vi "Main.vi"(8 "error in":errorcluster, 11 "ooxxMeter in":refnum<class "ooxxMeter.lvclass">) -> (0 "error out":errorcluster, 3 "ooxxMeter out":refnum<class "ooxxMeter.lvclass">)   [LabVIEW 2024, in "ooxxMeter.lvclass"]
doc: "The <b>Queued Message Handler</b> of the Worker that owns this VI."
uses:
  ooxxMeter.lvclass
  Initialization Data.ctl
  Response Cases.ctl
  <vilib>/addons/_Workers/Library/Case Label.ctl
  ooxxMeter.lvclass/ooxxMeter.ctl
  rql_MeterReadLoop.ctl
  rql_UpdatePanelDisplay.ctl
  rwr_ReadMeterValueNow.ctl
  rwr_ReadMeterValueNow Reply.ctl
  rqp_ReadValueAvg.ctl
  rsp_ReturnValueAvg.ctl
  <vilib>/numeric/Random Number (Range) DBL.vi
  20c30a35-eba6-49d0-a73b-0a0021e1c17a.vi
  <vilib>/Analysis/baseanly.llb/Mean (DBL).vi
  <vilib>/addons/_Workers/Library/Workers.lvlib
  <vilib>/Analysis/NI_AALBase.lvlib
panel:
  out "Meter":dbl(knob) scale=0.0..100.0
  out "ProgressBar":u8(slide) scale=0.0..100.0
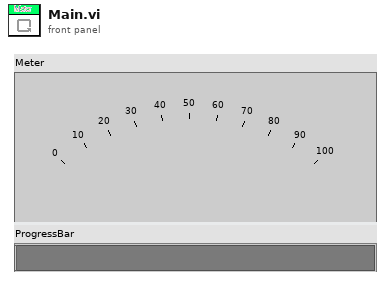
[diagram p1: front panel]
types:
  T1 = typedef "ooxxMeter.lvclass/Initialization Data.ctl" = cluster{"Response Cases":T2}
  T2 = typedef "ooxxMeter.lvclass/Response Cases.ctl" = cluster{"Placeholder - Can be deleted":string, "ReturnValueAvg":T3}
  T3 = typedef "Workers.lvlib/Case Label.ctl" = string
  T4 = typedef "ooxxMeter.lvclass/rql_MeterReadLoop.ctl" = cluster{"String":string}
  T5 = typedef "ooxxMeter.lvclass/rql_UpdatePanelDisplay.ctl" = cluster{"String":string}
  T6 = typedef "ooxxMeter.lvclass/rwr_ReadMeterValueNow Reply.ctl" = cluster{"String":string, "MeterValue":dbl}
  T7 = typedef "ooxxMeter.lvclass/rwr_ReadMeterValueNow.ctl" = cluster{"String":string}
  T8 = typedef "ooxxMeter.lvclass/rsp_ReturnValueAvg.ctl" = cluster{"String":string, "ValueAvg":dbl}
  T9 = typedef "ooxxMeter.lvclass/rqp_ReadValueAvg.ctl" = cluster{"String":string}
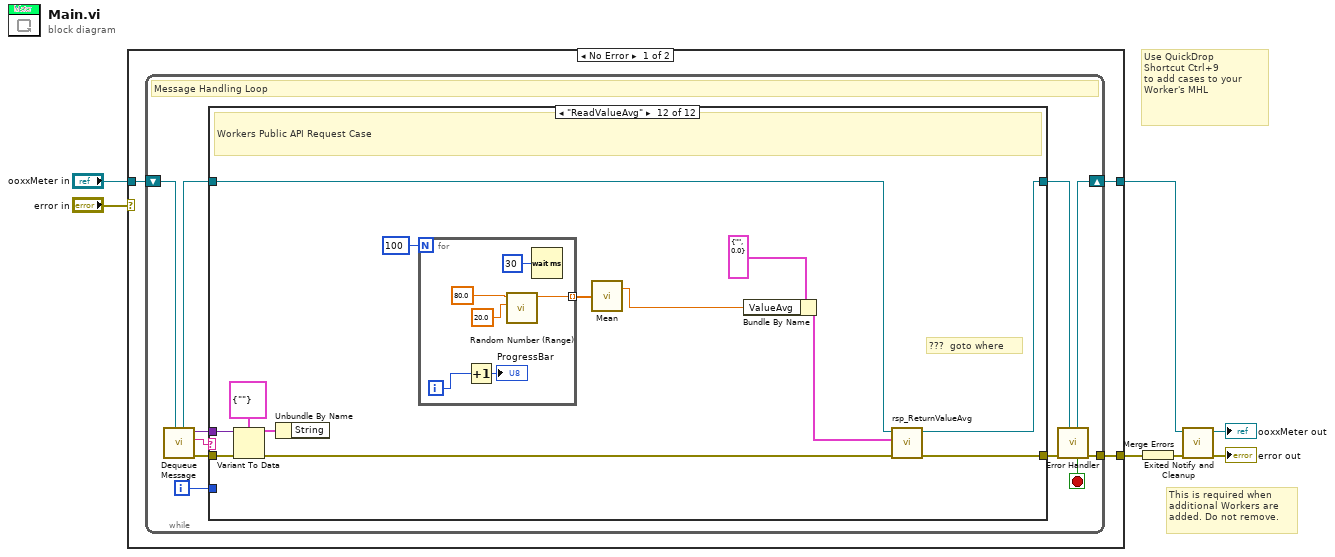
[diagram p0: block diagram]
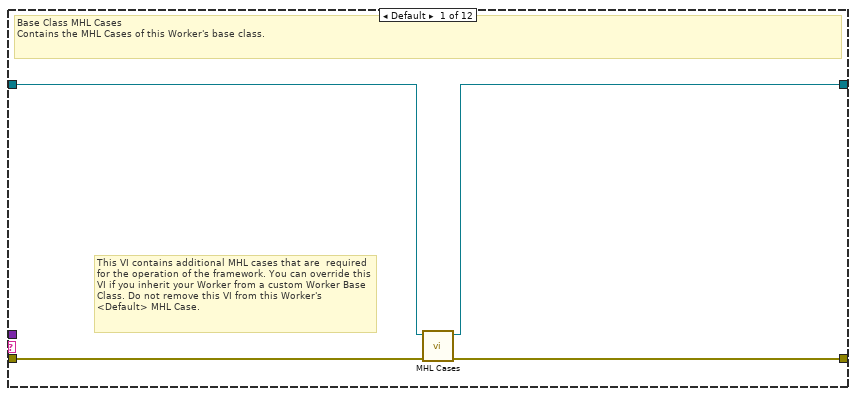
[diagram p2: hidden frame]
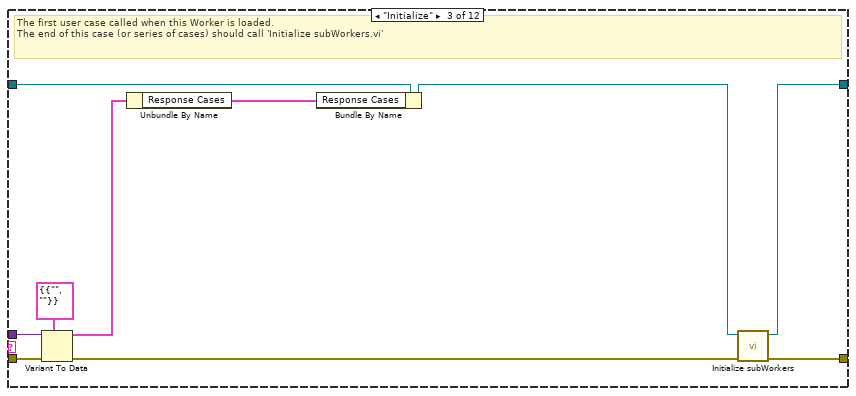
[diagram p4: hidden frame]
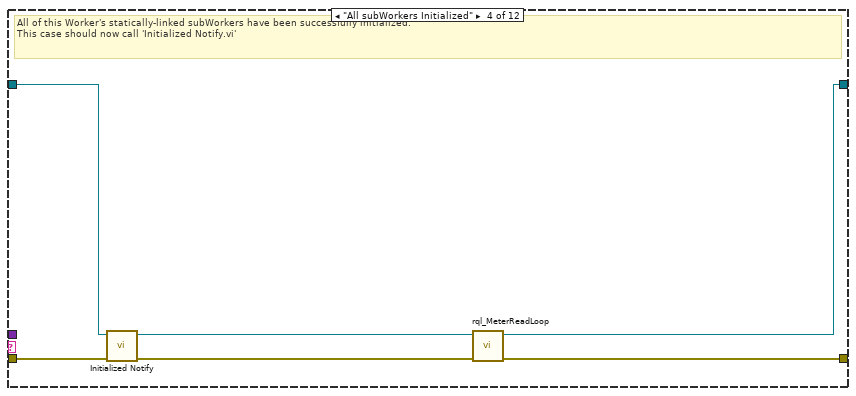
[diagram p5: hidden frame]
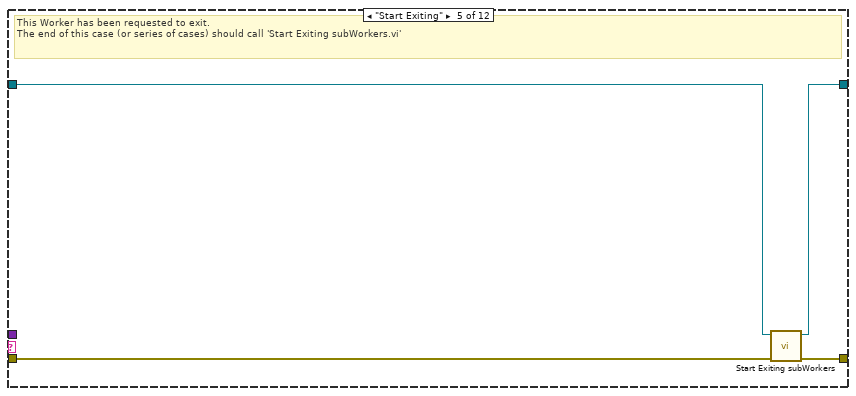
[diagram p6: hidden frame]
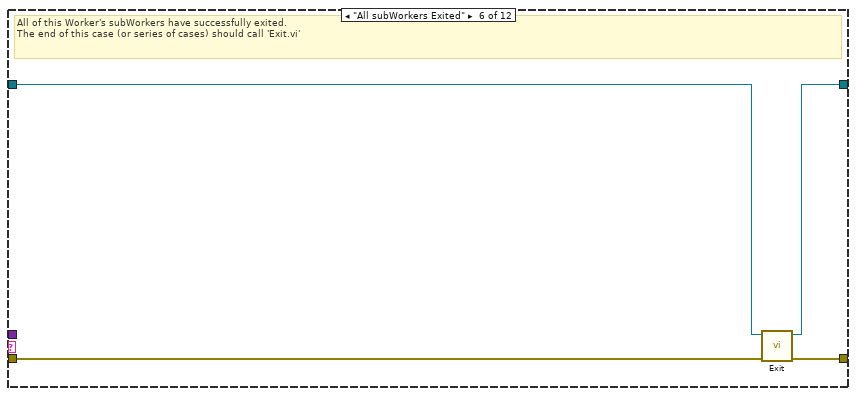
[diagram p7: hidden frame]
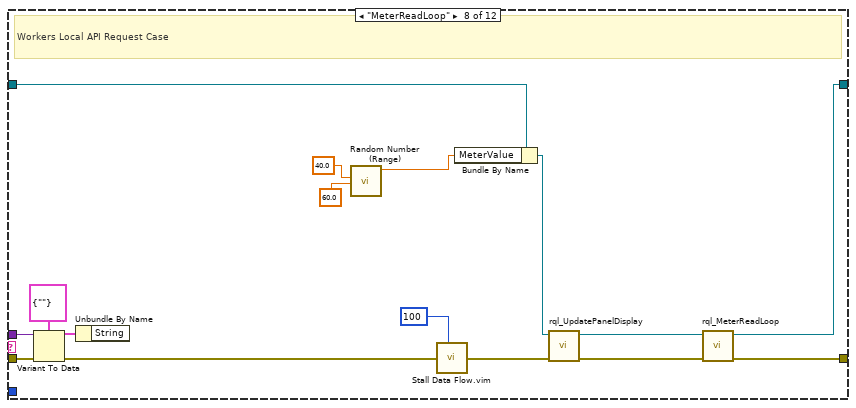
[diagram p9: hidden frame]
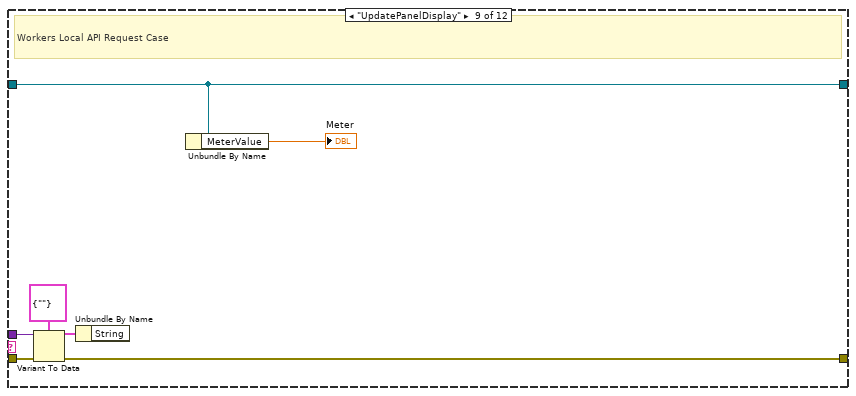
[diagram p10: hidden frame]
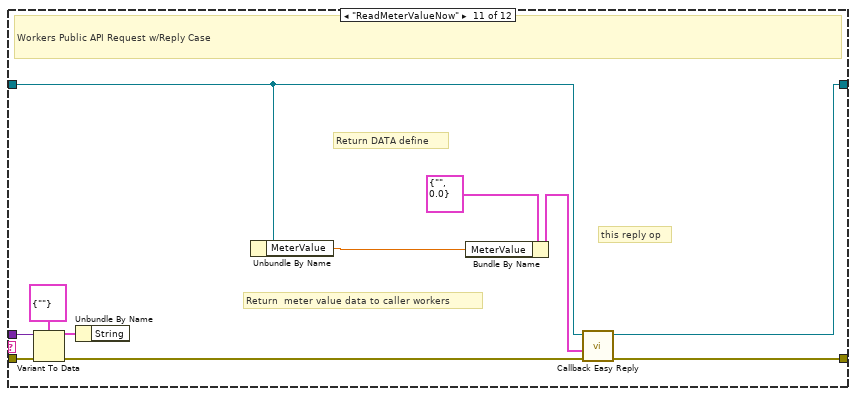
[diagram p12: hidden frame]
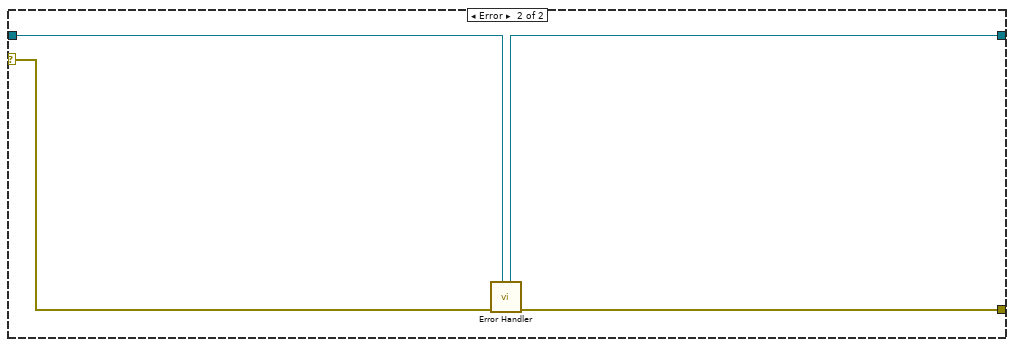
[diagram p13: hidden frame]
diagram:
  # "Use QuickDrop\nShortcut Ctrl+9\nto add cases to your\nWorker's MHL"
  # "This is required when additional Workers are added. Do not remove."
  n1 = case shown="No Error" "error in" {
    tunnel: "ooxxMeter in" -> [w8 w110]
    tunnel: [w10 w111] -> w6
    tunnel: [w9 w109] -> w7
    selector: "error in" -> [_ w112]
    frame No Error {
      n2 = while {
        shift-right: [w19] -> w9
        shift-left: w8 -> [w21]
        tunnel: [w20] -> w10
        i -> [w12]
        stop <- w13 stop-if-true
        # "Message Handling Loop"
        n3 = call-dynamic "Dequeue Message.vi"("Worker"=w21) -> ("error out"=w18:errorcluster, "Case out"=w14:string, "Data out"=w11:variant, "Worker out"=w16:refnum<class "ooxxMeter.lvclass">)  [unwired: 6 in, 1 out]
        n4 = case "Worker MHL Case Structure (DO NOT CHANGE LABEL NAME)" shown="\"ReadValueAvg\"" w14 {
          tunnel: w18 -> [w25 w26 w35 w43 w44 w51 w53 w68 w76 w78 w89 w102]
          tunnel: [w24 w26 w37 w40 w47 w50 w53 w56 w75 w78 w84 w95] -> w17
          tunnel: w16 -> [w23 w27 w34 w41 w45 w49 w52 w69 w71 w77 w80 w94]
          tunnel: [w22 w27 w36 w38 w46 w48 w52 w54 w71 w77 w83 w93] -> w15
          tunnel: w12 -> [_ _ _ _ _ _ _ _ _ _ _ _]
          tunnel: w11 -> [_ _ w32 _ _ _ _ w65 w73 _ w86 w99]
          frame Default {
            # "This VI contains additional MHL cases that are  required for the operation of the framework. You can override this VI if you inherit your Worker from a custom Worker Base Class. Do not remove this VI from this Worker's <Default> MHL Case."
            # "Base Class MHL Cases\nContains the MHL Cases of this Worker's base class."
            n5 = call-dynamic "MHL Cases.vi"("error in"=w25, "Worker in"=w23) -> ("error out"=w24:errorcluster, "Worker out"=w22:refnum<class "ooxxMeter.lvclass">)  [unwired: 8 in]
          }
          frame "------------ FRAMEWORK CASES -----------" {
            # "Start of Workers Framework Cases"
          }
          frame "Initialize" {
            # "The first user case called when this Worker is loaded.\nThe end of this case (or series of cases) should call 'Initialize subWorkers.vi'"
            n6 = Variant To Data(error in=w35, type=T1 {"Response Cases"={"Placeholder - Can be deleted"="", "ReturnValueAvg"=""}} ("Cluster"), Variant=w32) -> (data=w30:T1, error out=w33:errorcluster)
            n7 = Unbundle By Name(w30) -> ("Response Cases"=w29:T2)
            n8 = Bundle By Name(cluster=w34, "Response Cases"=w29) -> (w31:refnum<class "ooxxMeter.lvclass">)
            n9 = call-dynamic "Initialize subWorkers.vi"("error in"=w33, "Worker"=w31) -> ("error out"=w37:errorcluster, "dup Worker out"=w36:refnum<class "ooxxMeter.lvclass">)  [unwired: 8 in]
          }
          frame "All subWorkers Initialized" {
            # "All of this Worker's statically-linked subWorkers have been successfully initialized.\nThis case should now call 'Initialized Notify.vi'"
            n10 = call-dynamic "Initialized Notify.vi"("error in"=w43, "Worker"=w41) -> ("error out"=w42:errorcluster, "dup Worker out"=w39:refnum<class "ooxxMeter.lvclass">)  [unwired: 8 in]
            n11 = call "rql_MeterReadLoop.vi"("error in"=w42, "ooxxMeter in"=w39) -> ("error out"=w40:errorcluster, "dup ooxxMeter out"=w38:refnum<class "ooxxMeter.lvclass">)  [unwired: 8 in]
          }
          frame "Start Exiting" {
            # "This Worker has been requested to exit. \nThe end of this case (or series of cases) should call 'Start Exiting subWorkers.vi'"
            n12 = call-dynamic "Start Exiting subWorkers.vi"("error_in"=w44, "Worker"=w45) -> ("error out"=w47:errorcluster, "dup Worker out"=w46:refnum<class "ooxxMeter.lvclass">)  [unwired: 8 in]
          }
          frame "All subWorkers Exited" {
            # "All of this Worker's subWorkers have successfully exited. \nThe end of this case (or series of cases) should call 'Exit.vi'"
            n13 = call-dynamic "Exit.vi"("error_in"=w51, "Worker"=w49) -> ("error out"=w50:errorcluster, "dup Worker out"=w48:refnum<class "ooxxMeter.lvclass">)  [unwired: 8 in]
          }
          frame "------------- LOCAL API CASES -------------" {
            # "Start of Workers Local API Cases"
          }
          frame "MeterReadLoop" {
            # "Workers Local API Request Case"
            n14 = Variant To Data(error in=w68, type=T4 {"String"=""} ("Data"), Variant=w65) -> (data=w64:T4, error out=w67:errorcluster)
            n15 = Unbundle By Name(w64) -> ()  [unwired: 1 out]
            n16 = call-poly <vilib>:"Random Number (Range).vi"("lower bound (0)"=40.0, "upper bound (100)"=60.0) -> ("number"=w59:dbl)  [unwired: 9 in]
            n17 = call "Stall Data Flow.vim"("value in"=w67, "milliseconds to wait"=u32 100) -> ("value out"=w61:errorcluster)  [unwired: 1 out]
            n18 = Bundle By Name(cluster=w69, "MeterValue"=w59) -> (w57:refnum<class "ooxxMeter.lvclass">)
            n19 = call "rql_UpdatePanelDisplay.vi"("error in"=w61, "ooxxMeter in"=w57) -> ("error out"=w58:errorcluster, "dup ooxxMeter out"=w55:refnum<class "ooxxMeter.lvclass">)  [unwired: 8 in]
            n20 = call "rql_MeterReadLoop.vi"("error in"=w58, "ooxxMeter in"=w55) -> ("error out"=w56:errorcluster, "dup ooxxMeter out"=w54:refnum<class "ooxxMeter.lvclass">)  [unwired: 8 in]
          }
          frame "UpdatePanelDisplay" {
            # "Workers Local API Request Case"
            n21 = Variant To Data(error in=w76, type=T5 {"String"=""} ("Data"), Variant=w73) -> (data=w72:T5, error out=w75:errorcluster)
            n22 = Unbundle By Name(w72) -> ()  [unwired: 1 out]
            n23 = Unbundle By Name(w71) -> ("MeterValue"=→"Meter":dbl)
          }
          frame "------------- PUBLIC API CASES -------------" {
            # "Start of Workers Public API Cases"
          }
          frame "ReadMeterValueNow" {
            # "Return  meter value data to caller workers"
            # "Return DATA define"
            # "this reply op"
            # "Workers Public API Request w/Reply Case"
            n24 = Variant To Data(error in=w89, type=T7 {"String"=""} ("Data"), Variant=w86) -> (data=w85:T7, error out=w88:errorcluster)
            n25 = Unbundle By Name(w85) -> ()  [unwired: 1 out]
            n26 = Unbundle By Name(w80) -> ("MeterValue"=w79:dbl)
            n27 = Bundle By Name(cluster=T6 {"String"="", "MeterValue"=0.0} ("Reply Data"), "MeterValue"=w79) -> (w81:T6)
            n28 = call-dynamic "Callback Easy Reply.vi"("error in"=w88, "Data"=w81, "Worker"=w80) -> ("error out"=w84:errorcluster, "dup Worker out"=w83:refnum<class "ooxxMeter.lvclass">)  [unwired: 7 in]
          }
          frame "ReadValueAvg" {
            # "???  goto where"
            # "Workers Public API Request Case"
            n29 = Variant To Data(error in=w102, type=T9 {"String"=""} ("Data"), Variant=w99) -> (data=w98:T9, error out=w101:errorcluster)
            n30 = Unbundle By Name(w98) -> ()  [unwired: 1 out]
            n31 = for {
              N: 100 -> [_]
              tunnel: [w104] -> w96 mode=indexing
              i -> [w106]
              n32 = Increment(x=w106) -> (x+1=→"ProgressBar":i32)
              n33 = call-poly <vilib>:"Random Number (Range).vi"("lower bound (0)"=20.0, "upper bound (100)"=80.0) -> ("number"=w104:dbl)  [unwired: 9 in]
              n34 = Wait (ms)(milliseconds to wait=u32 30) -> ()  [unwired: 1 out]
            }
            n35 = call-poly <vilib>:"Mean.vi"("X"=w96) -> ("mean"=w90:dbl)  [unwired: 1 out]
            n36 = Bundle By Name(cluster=T8 {"String"="", "ValueAvg"=0.0} ("Data in"), "ValueAvg"=w90) -> (w91:T8)
            n37 = call "rsp_ReturnValueAvg.vi"("error in"=w101, "Data in"=w91, "ooxxMeter in"=w94) -> ("error out"=w95:errorcluster, "dup ooxxMeter out"=w93:refnum<class "ooxxMeter.lvclass">)  [unwired: 7 in]
          }
        }
        n38 = call-dynamic "Error Handler.vi"("Worker"=w15, "error_in"=w17) -> ("error out"=w20:errorcluster, "Stop Loop"=w13:bool, "Worker out"=w19:refnum<class "ooxxMeter.lvclass">)  [unwired: 7 in]
      }
    }
    frame Error {
      n39 = call-dynamic "Error Handler.vi"("Worker"=w110, "error_in"=w112) -> ("error out"=w111:errorcluster, "Worker out"=w109:refnum<class "ooxxMeter.lvclass">)  [unwired: 7 in, 1 out]
    }
  }
  n40 = Merge Errors(w6) -> (w3:errorcluster)
  n41 = call-dynamic "Exited Notify and Cleanup.vi"("error_in"=w3, "Worker"=w7) -> ("error out"=→"error out":errorcluster, "dup Worker out"=→"ooxxMeter out":refnum<class "ooxxMeter.lvclass">)  [unwired: 8 in]
